vi "selectXMLToConvert.vi"(11 "Sequence Context In":refnum<k7>) -> (0 "error out":errorcluster, 2 "DialogCancelled":bool, 3 "Selected Path":string)   [LabVIEW 2011]
doc: "Open the file dialog to allow the user to select an XML file to parse."
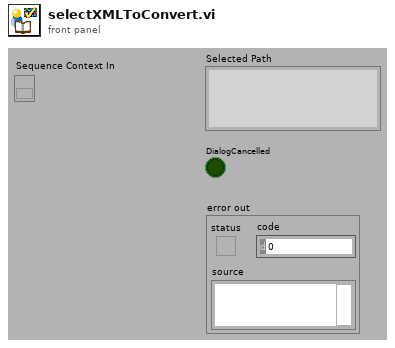
[diagram p1: front panel]
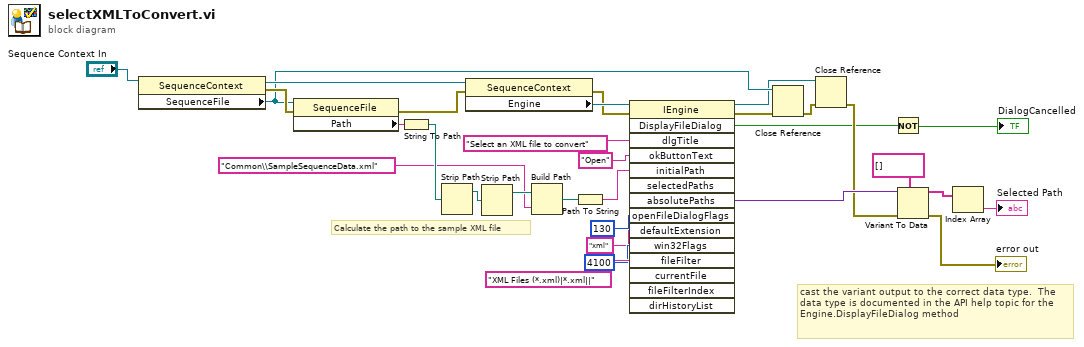
[diagram p0: block diagram]
diagram:
  # "cast the variant output to the correct data type.  The data type is documented in the API help topic for the Engine.DisplayFileDialog method"
  # "Calculate the path to the sample XML file"
  n1 = property class="SequenceContext"(reference="Sequence Context In") -> (reference out=w25:refnum<k7>, error out=w24:errorcluster, "SequenceFile"=w15:refnum<k7>)  [unwired: 1 in]
  n2 = property class="SequenceFile"(reference=w15, error in=w24) -> (error out=w26:errorcluster, "Path"=w23:string)  [unwired: 1 out]
  n3 = String To Path(string=w23) -> (path=w22:path)
  n4 = Strip Path(path=w22) -> (stripped path=w21:path)  [unwired: 1 out]
  n5 = property class="SequenceContext"(reference=w25, error in=w26) -> (error out=w30:errorcluster, "Engine"=w31:refnum<k7>)  [unwired: 1 out]
  n6 = Strip Path(path=w21) -> (stripped path=w20:path)  [unwired: 1 out]
  n7 = Build Path(base path=w20, name or relative path="Common\\SampleSequenceData.xml") -> (appended path=w18:path)
  n8 = Path To String(path=w18) -> (string=w3:string)
  n9 = invoke class="IEngine" method="DisplayFileDialog"(reference=w31, error in=w30, "dlgTitle"="Select an XML file to convert", "okButtonText"="Open", "initialPath"=w3, "openFileDialogFlags"=130, "defaultExtension"="xml", "win32Flags"=4100, "fileFilter"="XML Files (*.xml)|*.xml||") -> (reference out=w13:refnum<k7>, error out=w16:errorcluster, "DisplayFileDialog"=w2:bool, "absolutePaths"=w6:variant)  [unwired: 6 in, 11 out]
  n10 = Close Reference(reference=w15, error in (no error)=w16) -> (error out=w14:errorcluster)
  n11 = Close Reference(reference=w13, error in (no error)=w14) -> (error out=w5:errorcluster)
  n12 = Not(x=w2) -> (.not. x?=→"DialogCancelled":bool)
  n13 = Variant To Data(error in=w5, type=string[] [], Variant=w6) -> (data=w11:string[], error out=→"error out":errorcluster)
  n14 = Index Array(array=w11) -> (element=→"Selected Path":string)  [unwired: 1 in]
